vi "CPP-AQ.vi"() -> (5 "Plug in titles":string[](array[string]), 7 "Plug in values":string[](array[string]))   [LabVIEW 2020]
uses:
  Globals/Meas_global.vi
  CPPSW/CPP Global.vi
  <vilib>/Utility/miscctls.llb/LVPositionTypeDef.ctl
  <vilib>/Utility/miscctls.llb/LVForegroundBackgroundColorsTypeDef.ctl
panel:
  in  "Tab Control":enum32{"FID Traces", "Numerics"}(tab)
  out "FID Means":T1(graph)
  out "FID PPM":cluster{"Time (s)":dbl[], "Eng Values":dbl[]}[](graph)
  out "COV(%)":dbl[](array[numeric])
  out "sigma(ppm)":dbl[](array[numeric])
  out "DeltaMean(ppm)":dbl[](array[numeric])
  in  "Blocks":i32
  out "FIDsymbol":string[](array[string])
  out "PPM":dbl[](array[numeric]) format="%.1f"
  # "(Avg PPM Above BG)"
  # "https://en.wikipedia.org/wiki/Coefficient_of_variation"
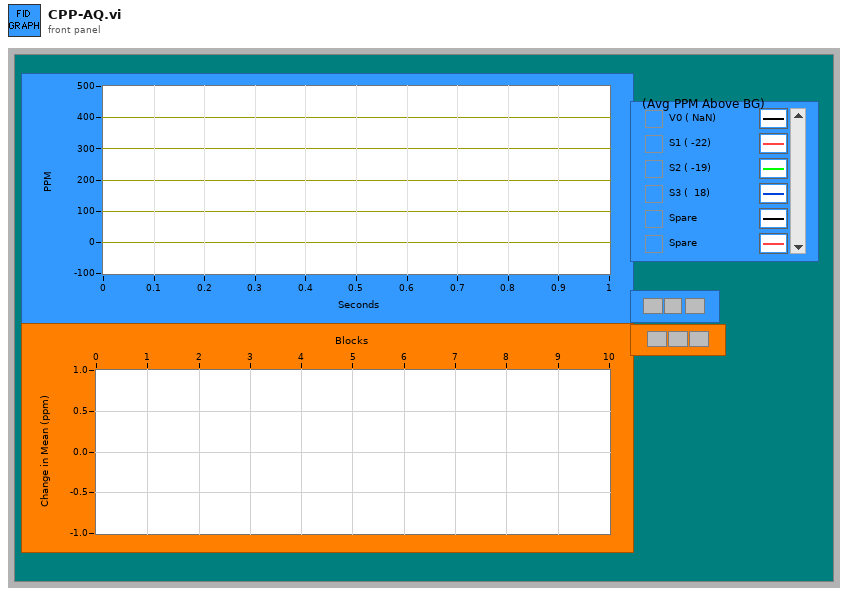
[diagram p1: front panel]
types:
  T1 = cluster{"[0]":dbl, "[1]":dbl, "[2]":dbl, "[3]":dbl}
  T2 = typedef "Analysis_info_cluster.ctl" = cluster{"Colour":u32, "Inst type":T3, "Inst name":string, "Symbol":string, "Code name":string, "Extra Info":string, "Inst Array":T4, "Extra Titles":string[], "Extra Values":string[], "U":dbl, "u^2":dbl, "u^3":dbl, "u^4":dbl, "Skew_u":dbl, "Kurt_u":dbl, "Sd Error in Mean":dbl, "% u'/U":dbl, "X":dbl, "Y":dbl, "Z":dbl, "Timescale integral Estimate":dbl, "Sd Error in Variance":dbl, "Calib File":path, "Calib Constants":dbl[], "Output Position":bool, "Stats":enum16{"None", "Basic", "Full"}, "Av Sampling Rate":dbl, "Av No of Samples":dbl, "Total Meas Time (s)":dbl, "ADAM Ch Name":string, "Max value":dbl, "Min value":dbl, "Req Sample Rate Hz":dbl, "Sync Delay Time (s)":dbl, "Ch No":i16, "Device":string, "Use Latest Calib":bool, "Port":string, "Metadata Ch Names":string[], "Metadata Ch Values":string[], "Label":string}
  T3 = typedef "Inst_type.ctl" = enum16{"Propeller anemometer", "Raw voltage", "Pressure Transducer", "Pitot-static tube", "Hot wire", "Cross wire 1", "Cross wire 2", "Generic Linear", "Generic Polynomial", "Generic BackPoly", "Fast FID", "Thermocouple", "Cold wire", "Pulsed Wire", "LDA Vel", "LDA Tran time", "LDA Arr time", "Microphone"}
  T4 = typedef "Instrument_Array.ctl" = enum16{"PWA", "LDA", "Analogue"}
  T5 = typedef "Time_Trace_Cluster.ctl" = cluster{"Weighting":dbl[], "Time (s)":dbl[], "Voltage":dbl[], "Eng Values":dbl[]}
  T6 = cluster{"[0]":dbl, "[1]":dbl, "[2]":dbl, "[3]":dbl}[]
  T7 = typedef "FIDmapping.ctl" = cluster{"Run #":dbl, "Run Suffix":u16, "Receptor #":u16, "ReceptorID":u16, "FIDname":string, "Long\nRun?":bool}[]
  T8 = cluster{"Receptor IDs":string[], "Receptor Numbers":u16[]}
  T9 = cluster{"Run #":dbl, "Run Suffix":u16, "Receptor #":u16, "ReceptorID":u16, "FIDname":string, "Long\nRun?":bool}
  T10 = typedef "LVPositionTypeDef.ctl" = cluster{"Left":i32, "Top":i32}
  T11 = typedef "LVForegroundBackgroundColorsTypeDef.ctl" = cluster{"Foreground Color":u32, "Background Color":u32}
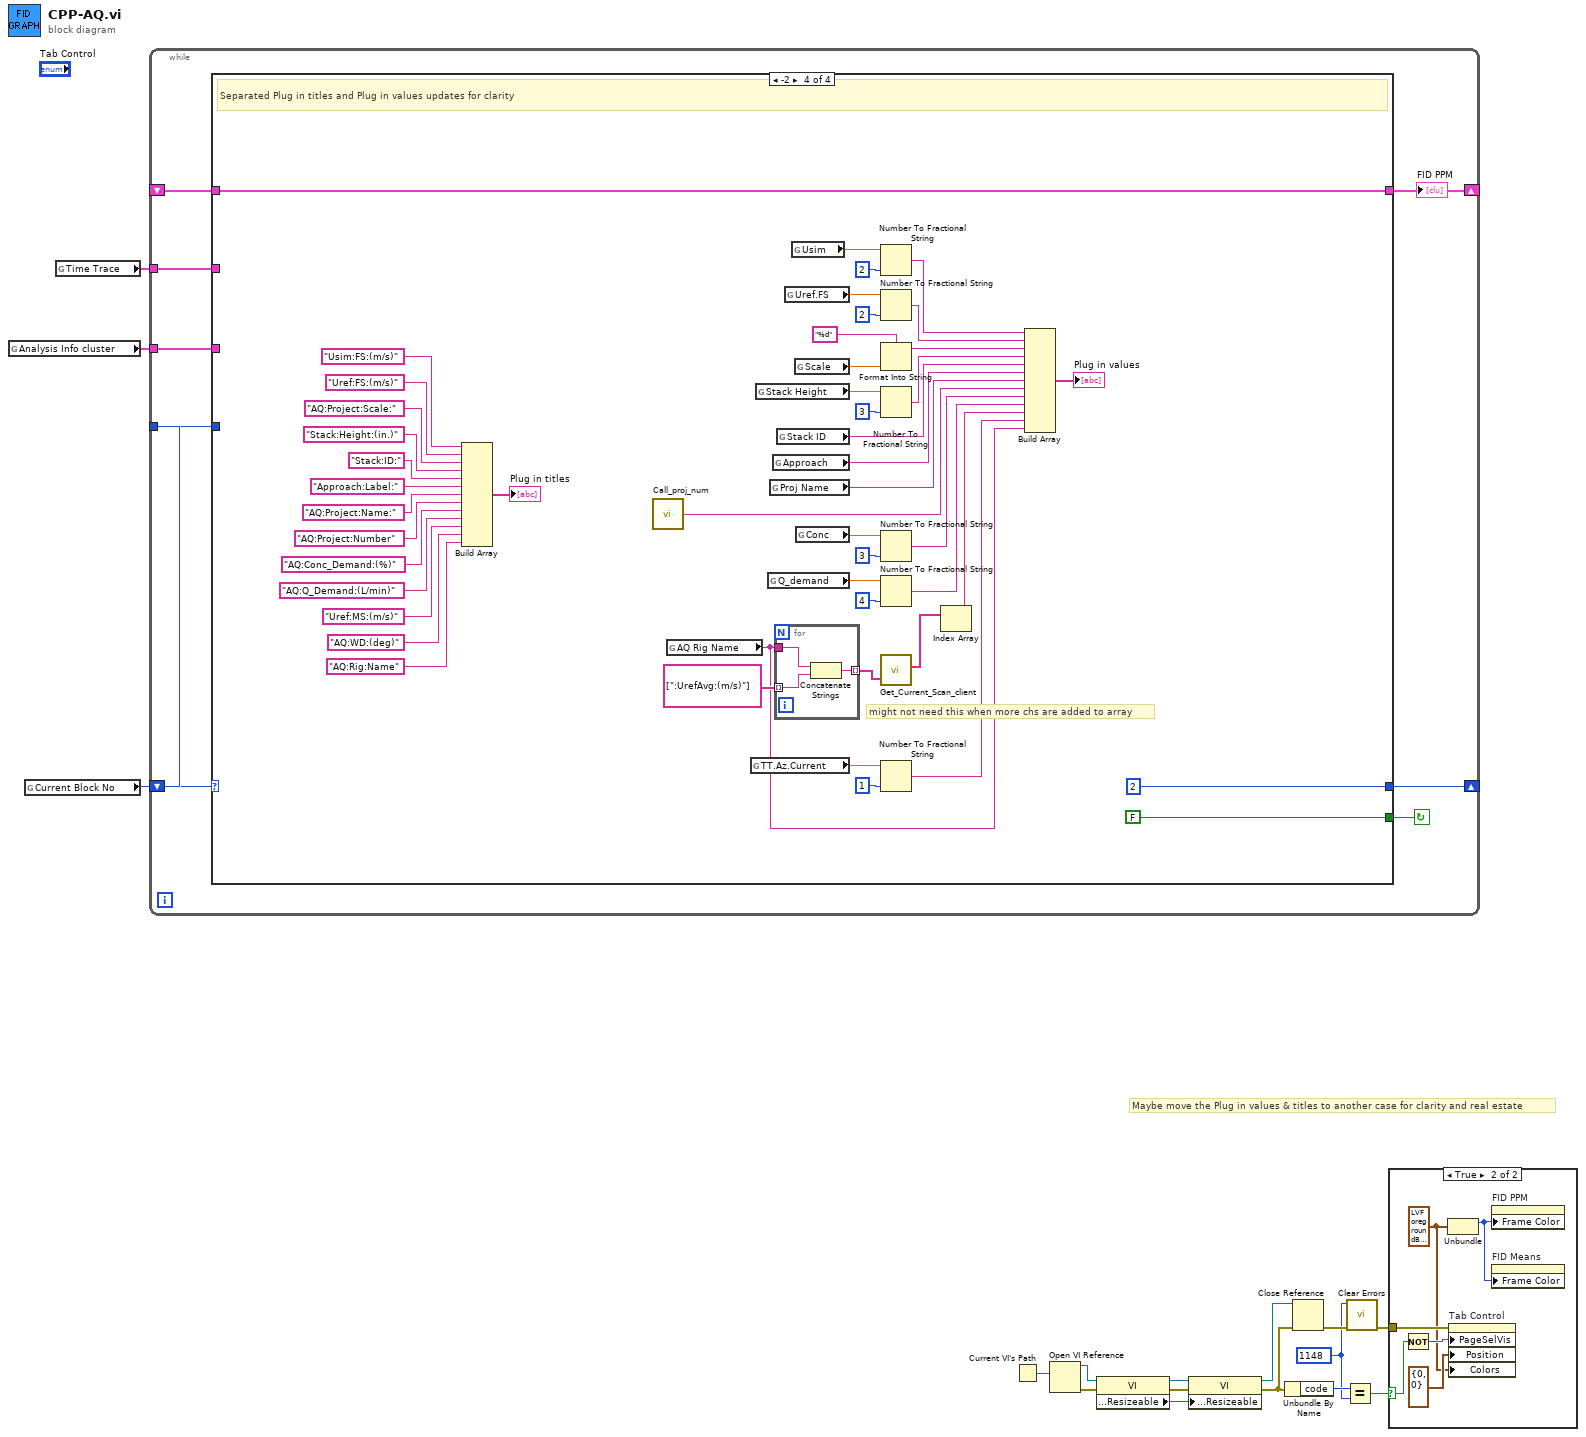
[diagram p0: block diagram]
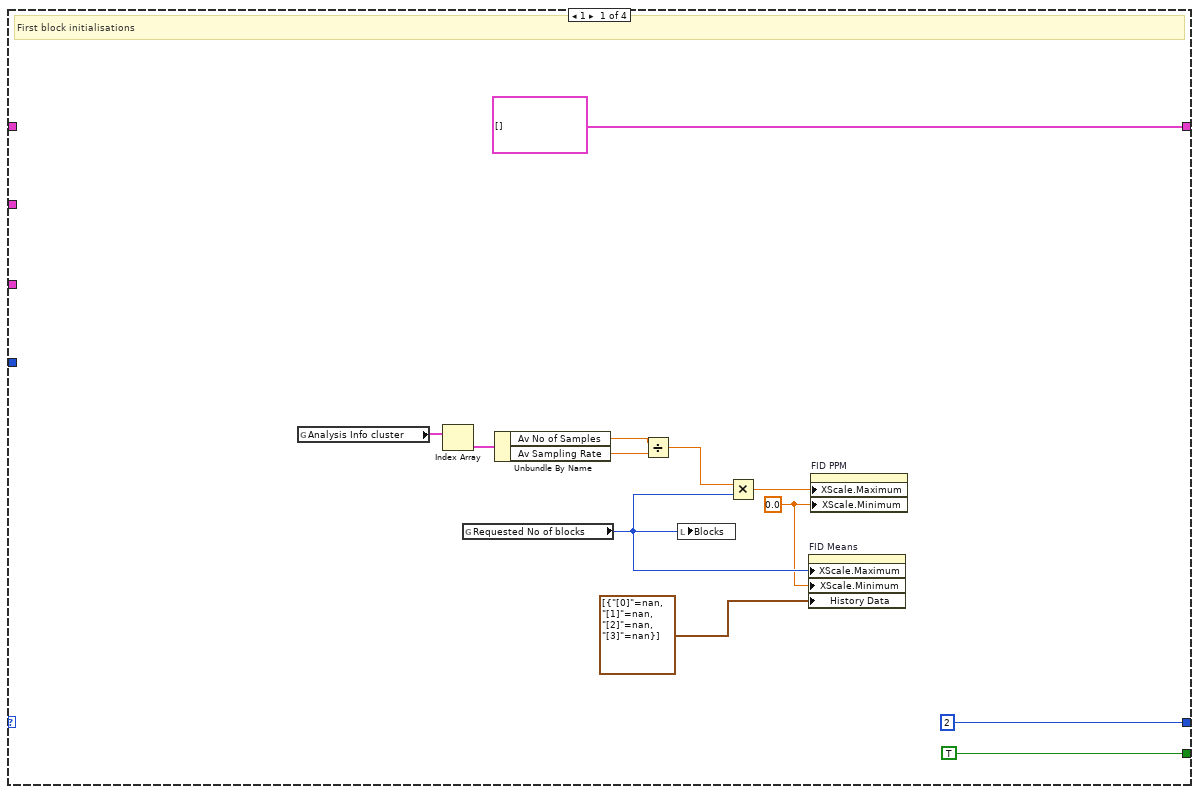
[diagram p3: hidden frame]
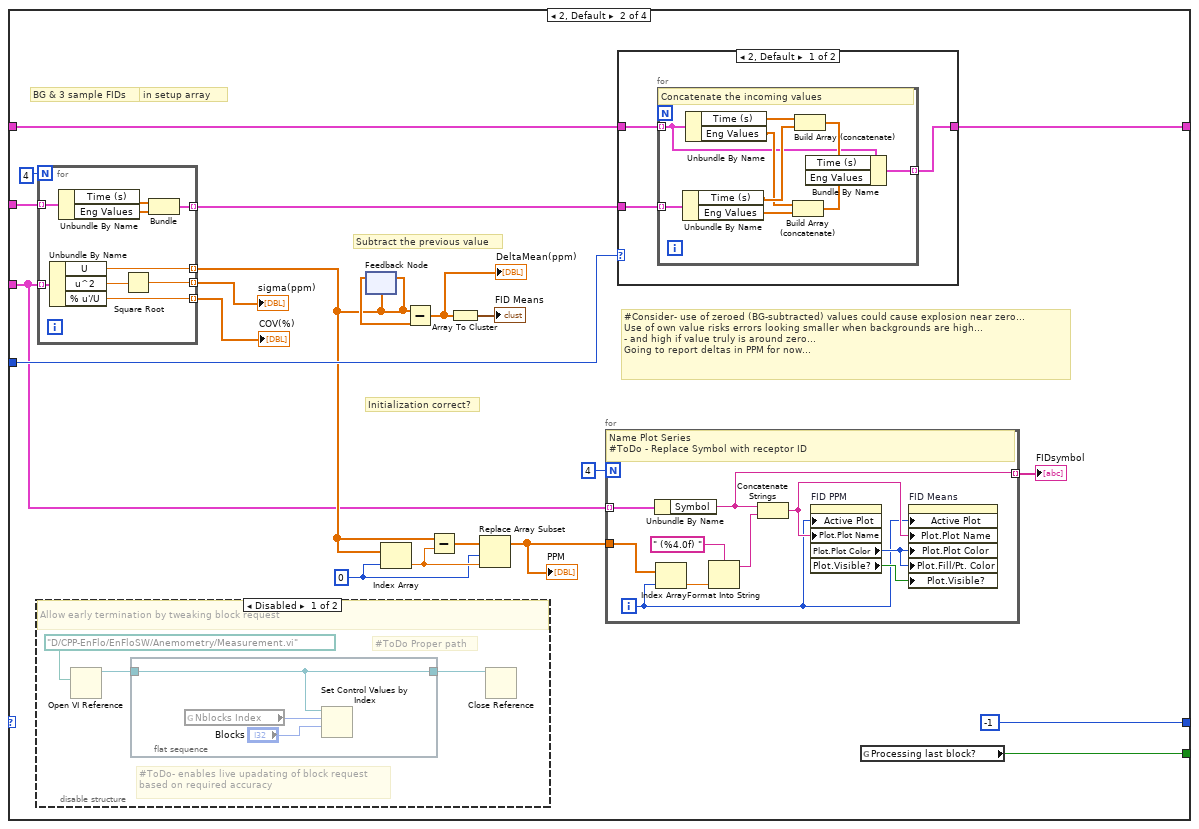
[diagram p4: hidden frame]
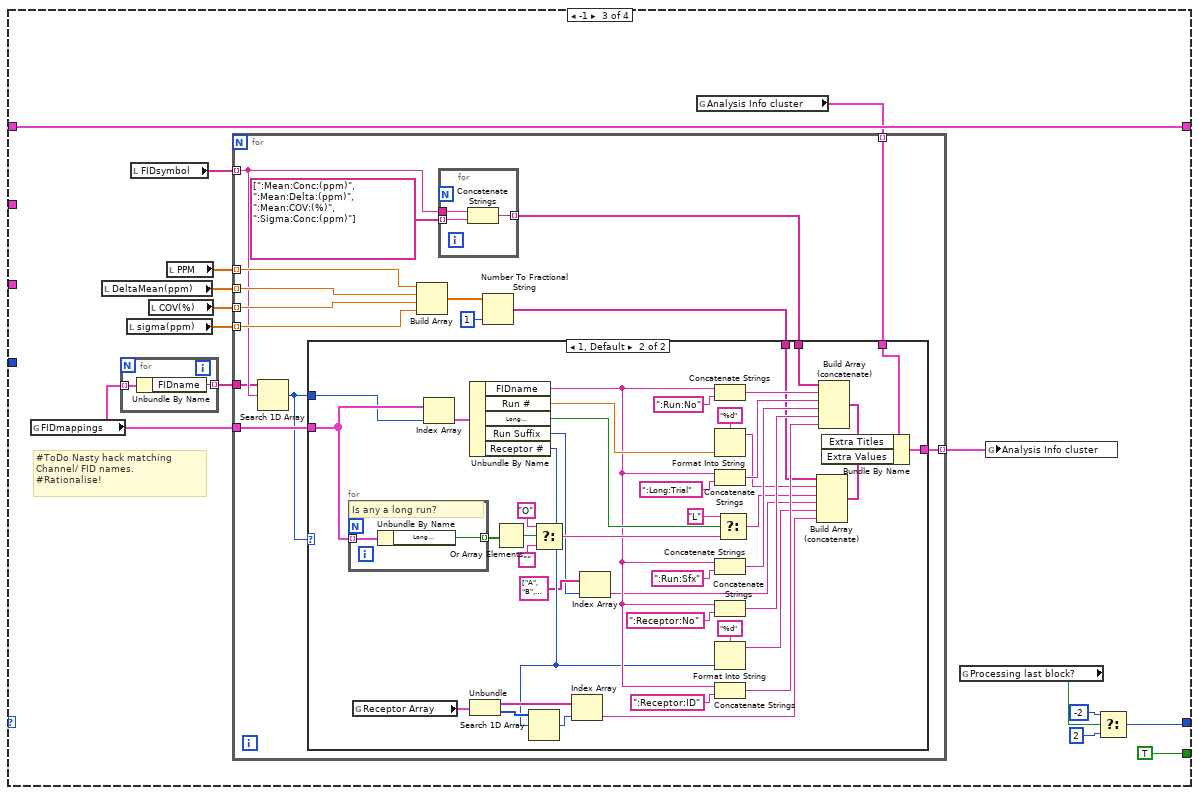
[diagram p7: hidden frame]
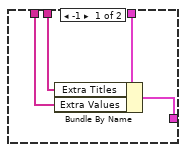
[diagram p8: hidden frame]
diagram:
  w3 = 1148 ("y")
  # "Maybe move the Plug in values & titles to another case for clarity and real estate"
  n1 = global read "Meas_global.vi" "Analysis Info cluster"() -> (w14:T2[])
  n2 = global read "Meas_global.vi" "Current Block No"() -> (w15:i32)
  n3 = global read "Meas_global.vi" "Time Trace"() -> (w16:T5[])
  n4 = while {
    shift-left: w15 -> [w21]
    shift-right: [w22] -> _
    tunnel: w16 -> [w23]
    tunnel: w15 -> [w20]
    tunnel: w14 -> [w19]
    shift-right: [w17] -> _
    shift-left: _ -> [w18]
    stop <- w24 continue-if-true
    n5 = case shown="-2" w21 {
      tunnel: [TRUE w56 TRUE FALSE ("Processing last block?")] -> w24
      tunnel: w23 -> [_ w57 _ _]
      tunnel: [2 -1 ("Case") w96 2 ("Case")] -> w22
      tunnel: w20 -> [_ w49 _ _]
      tunnel: w19 -> [_ w37 _ _]
      tunnel: [cluster{"Time (s)":dbl[], "Eng Values":dbl[]}[] [] w50 w109 w226] -> w17
      tunnel: w18 -> [_ w51 w109 w226]
      frame 1 {
        w25 = 0.0 ("X Scale.Range:Minimum")
        # "First block initialisations"
        n6 = global read "Meas_global.vi" "Analysis Info cluster"() -> (w28:T2[])
        n7 = Index Array(array=w28) -> (element=w29:T2)  [unwired: 1 in]
        n8 = global read "Meas_global.vi" "Requested No of blocks"() -> (w32:i32)
        n9 = Unbundle By Name(w29) -> ("Av No of Samples"=w30:dbl, "Av Sampling Rate"=w31:dbl)
        n10 = Divide(x=w30, y=w31) -> (x/y=w27:dbl)
        n11 = local write "Blocks"(w32) -> ()
        n12 = Multiply(x=w27, y=w32) -> (x*y=w34:dbl)
        n13 = property on="FID Means" class="WFChart (strict)"("XScale.Maximum"=w32, "XScale.Minimum"=w25, "History Data"=T6 [{"[0]"=nan, "[1]"=nan, "[2]"=nan, "[3]"=nan}]) -> ()  [unwired: 2 in, 2 out]
        n14 = property on="FID PPM" class="XYGraph (strict)"("XScale.Maximum"=w34, "XScale.Minimum"=w25) -> ()  [unwired: 2 in, 2 out]
      }
      frame 2, Default {
        w45 = 0 ("index")
        # "Initialization correct?"
        # "#Consider- use of zeroed (BG-subtracted) values could cause explosion near zero...\nUse of own value risks errors looking smaller when backgrounds are high...\n- and high if value truly is around zero...\nGoing to report deltas in PPM for now..."
        # "Subtract the previous value"
        # "BG FID is first element in setup array"
        # "BG & 3 sample FIDs"
        n15 = disable-structure shown="Disabled" {
          frame Disabled {
            # "#ToDo Proper path"
            # "#ToDo- enables live upadating of block request based on required accuracy"
            # "Allow early termination by tweaking block request"
            n16 = Open VI Reference(vi path=path "D:/CPP-EnFlo/EnFloSW/Anemometry/Measurement.vi") -> (vi reference=w59:refnum<vi>)  [unwired: 5 in, 1 out]
            n17 = flat-sequence {
              tunnel: w59 -> [w61]
              tunnel: [w61] -> w58
              frame #0 {
                n18 = global read "Meas_global.vi" "Nblocks Index"() -> (w63:i32)
                n19 = Set Control Values by Index(0:w61, 1:w63, 2:"Blocks") -> ()  [unwired: 1 in, 1 out]
              }
            }
            n20 = Close Reference(reference=w58) -> ()  [unwired: 1 in, 1 out]
          }
          frame Enabled {
          }
        }
        n21 = for {
          N: 4 -> [_]
          tunnel: w57 -> [w95] mode=indexing
          tunnel: w37 -> [w94] mode=indexing
          tunnel: [w93] -> w42 mode=indexing
          tunnel: [w90] -> w52 mode=indexing
          tunnel: [w88] -> w44 mode=indexing
          tunnel: [w87] -> w43 mode=indexing
          n22 = Unbundle By Name(w94) -> ("U"=w93:dbl, "u^2"=w89:dbl, "% u'/U"=w87:dbl)
          n23 = Unbundle By Name(w95) -> ("Time (s)"=w92:dbl[], "Eng Values"=w91:dbl[])
          n24 = Square Root(x=w89) -> (sqrt(x)=w88:dbl)
          n25 = Bundle("Time (s)"=w92, "Eng Values"=w91) -> (w90:cluster{"Time (s)":dbl[], "Eng Values":dbl[]})  [unwired: 1 in]
        }
        "sigma(ppm)" <- w44
        "COV(%)" <- w43
        n26 = feedback-in #1(w42) -> ()
        n27 = feedback #1(w42) -> (w53:dbl[])
        n28 = Index Array(array=w42, index=w45) -> (element=w46:dbl)
        n29 = Subtract(x=w42, y=w53) -> (x-y=w41:dbl[])
        "DeltaMean(ppm)" <- w41
        n30 = Subtract(x=w42, y=w46) -> (x-y=w47:dbl[])
        n31 = Array To Cluster(array=w41) -> (cluster=→"FID Means":T1)
        n32 = Replace Array Subset(array=w47, new element=w46, index=w45) -> (w38:dbl[])
        "PPM" <- w38
        n33 = for {
          N: 4 -> [_]
          tunnel: w37 -> [w73] mode=indexing
          tunnel: [w64] -> w39 mode=indexing
          tunnel: w38 -> [w67]
          i -> [w66]
          # "Name Plot Series\n#ToDo - Replace Symbol with receptor ID"
          n34 = Unbundle By Name(w73) -> ("Symbol"=w64:string)
          n35 = Index Array(array=w67, index=w66) -> (element=w65:dbl)
          n36 = Format Into String(format string=" (%4.0f) ", w65) -> (resulting string=w68:string)  [unwired: 2 in, 1 out]
          n37 = Concatenate Strings(w64, w68) -> (w70:string)
          n38 = property on="FID PPM" class="XYGraph (strict)"("Active Plot"=w66, "Plot.Plot Name"=w70) -> ("Plot.Plot Color"=w72:u32, "Plot.Visible?"=w71:bool)  [unwired: 2 in, 2 out]
          n39 = property on="FID Means" class="WFChart (strict)"("Active Plot"=w66, "Plot.Plot Name"=w70, "Plot.Plot Color"=w72, "Plot.Fill/Pt. Color"=w72, "Plot.Visible?"=w71) -> ()  [unwired: 2 in, 2 out]
        }
        "FIDsymbol" <- w39
        n40 = case shown="2, Default" w49 {
          tunnel: [w74 w86] -> w50
          tunnel: w52 -> [w76 w86]
          tunnel: w51 -> [w75 _]
          frame 2, Default {
            n41 = for {
              tunnel: w75 -> [w78] mode=indexing
              tunnel: w76 -> [w77] mode=indexing
              tunnel: [w79] -> w74 mode=indexing
              # "Concatenate the incoming values"
              n42 = Unbundle By Name(w77) -> ("Time (s)"=w84:dbl[], "Eng Values"=w83:dbl[])
              n43 = Unbundle By Name(w78) -> ("Time (s)"=w85:dbl[], "Eng Values"=w82:dbl[])
              n44 = Build Array (concatenate)(w82, w83) -> (w80:dbl[])
              n45 = Build Array (concatenate)(w85, w84) -> (w81:dbl[])
              n46 = Bundle By Name(cluster=w78, "Time (s)"=w81, "Eng Values"=w80) -> (w79:cluster{"Time (s)":dbl[], "Eng Values":dbl[]})
            }
          }
          frame 1 {
            # "Initialise with first block of data"
          }
        }
        n47 = global read "Meas_global.vi" "Processing last block?"() -> (w56:bool)
      }
      frame -1 {
        # "#ToDo Nasty hack matching Channel/ FID names.\n#Rationalise!"
        n48 = global read "CPP Global.vi" "FIDmappings"() -> (w101:T7)
        n49 = local read "DeltaMean(ppm)"() -> (w103:dbl[])
        n50 = for {
          tunnel: w101 -> [w112] mode=indexing
          tunnel: [w111] -> w100 mode=indexing
          n51 = Unbundle By Name(w112) -> ("FIDname"=w111:string)
        }
        n52 = local read "sigma(ppm)"() -> (w104:dbl[])
        n53 = local read "FIDsymbol"() -> (w108:string[])
        n54 = local read "COV(%)"() -> (w102:dbl[])
        n55 = local read "PPM"() -> (w105:dbl[])
        n56 = global read "Meas_global.vi" "Analysis Info cluster"() -> (w107:T2[])
        n57 = for {
          tunnel: w108 -> [w115] mode=indexing
          tunnel: w107 -> [w124] mode=indexing
          tunnel: [w123] -> w106 mode=indexing
          tunnel: w105 -> [w122] mode=indexing
          tunnel: w104 -> [w121] mode=indexing
          tunnel: w103 -> [w120] mode=indexing
          tunnel: w102 -> [w119] mode=indexing
          tunnel: w101 -> [w118]
          tunnel: w100 -> [w114]
          n58 = Search 1D Array(1D array=w114, element=w115) -> (index of element=w113:i32)  [unwired: 1 in]
          n59 = Build Array(w122, w120, w119, w121) -> (w127:dbl[])
          n60 = for {
            tunnel: w115 -> [w178]
            tunnel: string[] [":Mean:Conc:(ppm)", ":Mean:Delta:(ppm)", ":Mean:COV:(%)", ":Sigma:Conc:(ppm)"] -> [w177] mode=indexing
            tunnel: [w176] -> w117 mode=indexing
            n61 = Concatenate Strings(w178, w177) -> (w176:string)
          }
          n62 = Number To Fractional String(number=w127, precision (6)=i16 1) -> (F-format string=w116:string[])  [unwired: 2 in]
          n63 = case shown="1, Default" w113 {
            tunnel: w124 -> [w131 w173]
            tunnel: [w130 w172] -> w123
            tunnel: w118 -> [_ w150]
            tunnel: w117 -> [w129 w144]
            tunnel: w116 -> [w128 w139]
            tunnel: w113 -> [_ w135]
            frame -1 {
              n64 = Bundle By Name(cluster=w131, "Extra Titles"=w129, "Extra Values"=w128) -> (w130:T2)
            }
            frame 1, Default {
              n65 = for {
                tunnel: w150 -> [w175] mode=indexing
                tunnel: [w174] -> w171 mode=indexing
                # "Is any a long run?"
                n66 = Unbundle By Name(w175) -> ("Long\nRun?"=w174:bool)
              }
              n67 = global read "CPP Global.vi" "Receptor Array"() -> (w154:T8)
              n68 = Index Array(array=w150, index=w135) -> (element=w151:T9)
              n69 = Unbundle By Name(w151) -> ("FIDname"=w156:string, "Run #"=w165:dbl, "Long\nRun?"=w163:bool, "Run Suffix"=w133:u16, "Receptor #"=w136:u16)
              n70 = Unbundle(w154) -> ("Receptor IDs"=w152:string[], "Receptor Numbers"=w153:u16[])
              n71 = Or Array Elements(Boolean array=w171) -> (logical OR=w170:bool)
              n72 = Search 1D Array(1D array=w153, element=w136) -> (index of element=w155:i32)  [unwired: 1 in]
              n73 = Select(t="O" ("string"), s=w170, f="") -> (s? t:f=w167:string)
              n74 = Index Array(array=w152, index=w155) -> (element=w140:string)
              n75 = Index Array(array=string[] ["A", "B", "C", "D", "E", "F", "G", "H", "I", "J", "K", "L", "M", "N", "O", "P", "Q", "R", "S", "T", "U", "V", "W", "X", "Y", "Z"], index=w133) -> (element=w132:string)
              n76 = Concatenate Strings(w156, ":Run:No" ("string")) -> (w149:string)
              n77 = Format Into String(format string="%d", w165) -> (resulting string=w143:string)  [unwired: 2 in, 1 out]
              n78 = Concatenate Strings(w156, ":Long:Trial" ("string")) -> (w148:string)
              n79 = Concatenate Strings(w156, ":Run:Sfx" ("string")) -> (w147:string)
              n80 = Concatenate Strings(w156, ":Receptor:No" ("string")) -> (w146:string)
              n81 = Format Into String(format string="%d", w136) -> (resulting string=w141:string)  [unwired: 2 in, 1 out]
              n82 = Concatenate Strings(w156, ":Receptor:ID" ("string")) -> (w145:string)
              n83 = Select(t="L" ("string"), s=w163, f=w167) -> (s? t:f=w142:string)
              n84 = Build Array (concatenate)(w139, w143, w142, w132, w141, w140) -> (w137:string[])
              n85 = Build Array (concatenate)(w144, w149, w148, w147, w146, w145) -> (w138:string[])
              n86 = Bundle By Name(cluster=w173, "Extra Titles"=w138, "Extra Values"=w137) -> (w172:T2)
            }
          }
        }
        n87 = global read "Meas_global.vi" "Processing last block?"() -> (w99:bool)
        n88 = global write "Meas_global.vi" "Analysis Info cluster"(w106) -> ()
        n89 = Select(t=-2, s=w99, f=2 ("Case")) -> (s? t:f=w96:i32)
      }
      frame -2 {
        # "might not need this when more chs are added to array"
        # "Separated Plug in titles and Plug in values updates for clarity"
        n90 = Build Array("Usim:FS:(m/s)", "Uref:FS:(m/s)" ("element"), "AQ:Project:Scale:", "Stack:Height:(in.)", "Stack:ID:", "Approach:Label:", "AQ:Project:Name:", "AQ:Project:Number" ("element"), "AQ:Conc_Demand:(%)" ("element"), "AQ:Q_Demand:(L/min)" ("element"), "Uref:MS:(m/s)" ("element"), "AQ:WD:(deg)" ("element"), "AQ:Rig:Name" ("element")) -> (→"Plug in titles":string[])
        n91 = call "Call_proj_num.vi"() -> ("ProjectNumber"=w179:string)  [unwired: 1 in]
        n92 = global read "CPP Global.vi" "AQ Rig Name"() -> (w180:string)
        n93 = global read "CPP Global.vi" "TT.Az.Current"() -> (w184:dbl)
        n94 = global read "CPP Global.vi" "Stack Height"() -> (w203:dbl)
        n95 = global read "CPP Global.vi" "Q_demand"() -> (w190:dbl)
        n96 = global read "CPP Global.vi" "Proj Name"() -> (w196:string)
        n97 = global read "CPP Global.vi" "Approach"() -> (w200:string)
        n98 = for {
          tunnel: string[] [":UrefAvg:(m/s)"] -> [w229] mode=indexing
          tunnel: [w228] -> w188 mode=indexing
          tunnel: w180 -> [w227]
          n99 = Concatenate Strings(w227, w229) -> (w228:string)
        }
        n100 = global read "CPP Global.vi" "Stack ID"() -> (w201:string)
        n101 = global read "CPP Global.vi" "Uref.FS"() -> (w198:dbl)
        n102 = global read "CPP Global.vi" "Usim"() -> (w210:dbl)
        n103 = global read "CPP Global.vi" "Scale"() -> (w206:dbl)
        n104 = global read "CPP Global.vi" "Conc"() -> (w194:dbl)
        n105 = Number To Fractional String(number=w210, precision (6)=i16 2) -> (F-format string=w208:string)  [unwired: 2 in]
        n106 = Number To Fractional String(number=w198, precision (6)=i16 2) -> (F-format string=w197:string)  [unwired: 2 in]
        n107 = Format Into String(format string="%d", w206) -> (resulting string=w205:string)  [unwired: 2 in, 1 out]
        n108 = Number To Fractional String(number=w203, precision (6)=i16 3) -> (F-format string=w202:string)  [unwired: 2 in]
        n109 = Number To Fractional String(number=w194, precision (6)=i16 3) -> (F-format string=w193:string)  [unwired: 2 in]
        n110 = Number To Fractional String(number=w190, precision (6)=i16 4) -> (F-format string=w191:string)  [unwired: 2 in]
        n111 = call "Get_Current_Scan_client.vi"("multipleChannels"=w188) -> ("String values"=w186:string[])  [unwired: 2 in, 2 out]
        n112 = Number To Fractional String(number=w184, precision (6)=i16 1) -> (F-format string=w183:string)  [unwired: 2 in]
        n113 = Index Array(array=w186) -> (element=w187:string)  [unwired: 1 in]
        n114 = Build Array(w208, w197, w205, w202, w201, w200, w196, w179, w193, w191, w187, w183, w180) -> (→"Plug in values":string[])
      }
    }
    "FID PPM" <- w17
  }
  n115 = Current VI's Path() -> (path=w6:path)
  n116 = Open VI Reference(vi path=w6) -> (vi reference=w7:refnum<vi>, error out=w8:errorcluster)  [unwired: 5 in]
  n117 = property class="VI"(reference=w7, error in=w8) -> (reference out=w9:refnum<vi>, error out=w10:errorcluster, "Front Panel.Resizeable"=w11:bool)
  n118 = property class="VI"(reference=w9, error in=w10, "Front Panel.Resizeable"=w11) -> (reference out=w12:refnum<vi>, error out=w5:errorcluster)
  n119 = Unbundle By Name(w5) -> ("code"=w13:i32)
  n120 = Close Reference(reference=w12, error in (no error)=w5) -> (error out=w4:errorcluster)
  n121 = Equal?(x=w13, y=w3) -> (x = y?=w1:bool)
  n122 = call <vilib>:"Clear Errors.vi"("error in (no error)"=w4, "specific error code to clear (0: all)"=w3) -> ("error out"=w2:errorcluster)  [unwired: 4 in, 1 out]
  n123 = case shown="True" w1 {
    selector: w1 -> [_ w232]
    tunnel: w2 -> [_ w235]
    frame False {
    }
    frame True {
      w231 = T11 {"Foreground Color"=16738740, "Background Color"=16738740} ("Colors")
      n124 = Not(x=w232) -> (.not. x?=w234:bool)
      n125 = Unbundle(w231) -> ("Foreground Color"=w230:u32)  [unwired: 1 out]
      n126 = property on="Tab Control" class="TabCtl (strict)"(error in=w235, "PageSelVis"=w234, "Position"=T10 {"Left"=0, "Top"=0}, "Colors"=w231) -> ()  [unwired: 1 in, 2 out]
      n127 = property on="FID PPM" class="XYGraph (strict)"("Frame Color"=w230) -> ()  [unwired: 2 in, 2 out]
      n128 = property on="FID Means" class="WFChart (strict)"("Frame Color"=w230) -> ()  [unwired: 2 in, 2 out]
    }
  }
